vi "Ex1_Add.vi"() -> ()   [LabVIEW 2013]
uses:
  Add/codegen/dll/Ex1_add/Ex1_add.dll
panel:
  out "Sum":dbl
  in  "b":dbl
  in  "a":dbl
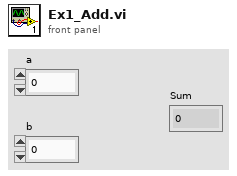
[diagram p1: front panel]
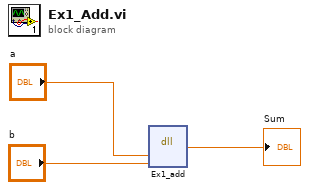
[diagram p0: block diagram]
diagram:
  n1 = dll-call lib="PTH1µabs D5-æ çº¿éä¿¡ä¹¦ç±ç¼å+åºäºLabVIEWçè½¯ä»¶æ çº¿çµå¥é¨æç¨ä¹¦ç±ç« èç¨åº6.ç¬¬å­ç« Exercise6.1-Add-DLL_X64AddcodegendllEx1_addEx1_add.dll" fn="Ex1_add"("a"="a", "b"="b") -> ("Sum"=→"Sum":dbl)  [unwired: 5 in, 2 out]
